vi "Periodic Tasks.vi"(8 "error in":errorcluster) -> ()   [LabVIEW 2018]
doc: "This VI runs in parallel to other robot code. It can contain as many user-defined periodic loops as you need. These can carry out PID or other sorts of timed response."
panel:
  in  "Seconds from neutral to full (0)":sgl=0.08
  out "Transmit FIFO Full Count":u32
  out "Bus Off Count":u32
  out "Percent Bus Utilization":sgl
  out "Receive Error Count":u32
  out "Transmit Error Count":u32
  out "error out":errorcluster
  in  "error in (no error)":errorcluster
  out "Waveform Chart 3":T1(graph)
  out "Waveform Chart 2":T2(graph)
  out "Waveform Chart":dbl(graph)
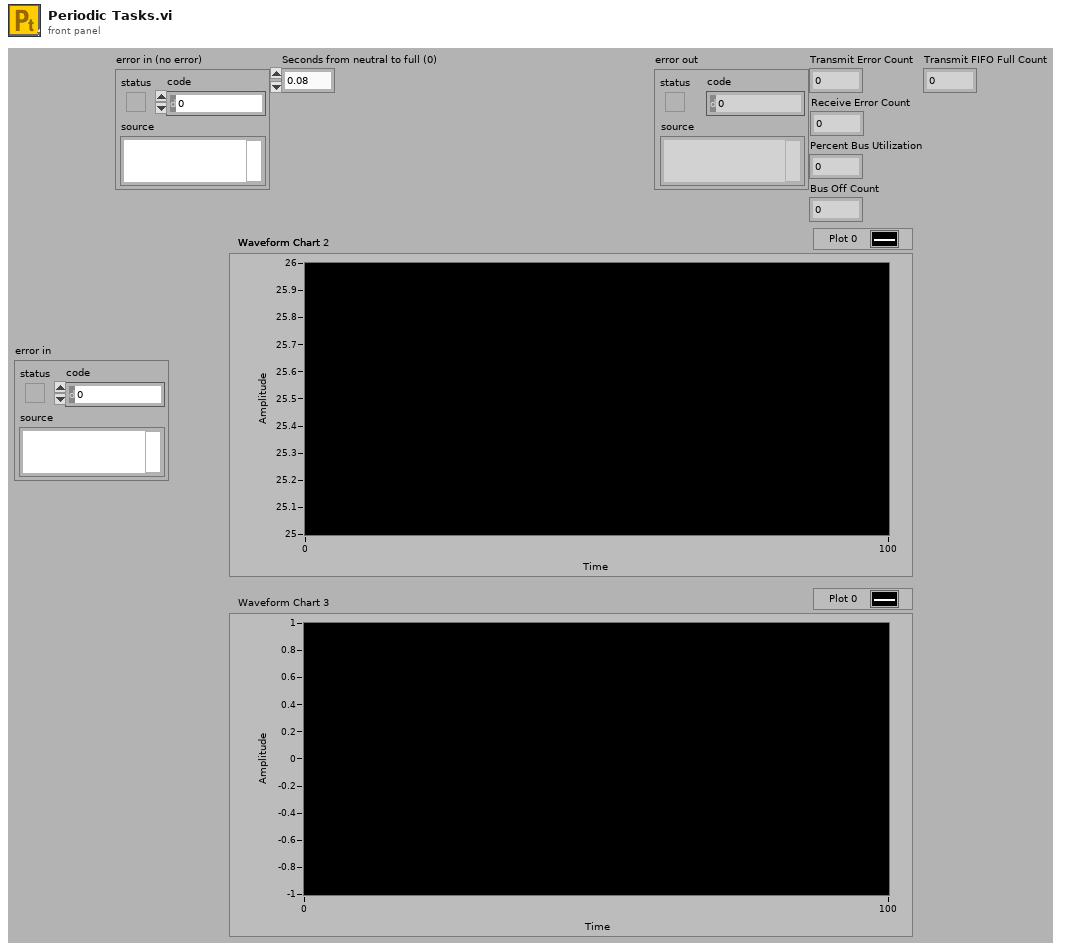
[diagram p1: front panel]
types:
  T1 = cluster{"Sensor Velocity":dbl, "Sensor Velocity":dbl, "Sensor Velocity":dbl}
  T2 = cluster{"Motor Temperature":u8, "Motor Temperature":u8, "Motor Temperature":u8}
  T3 = typedef "SPARKMAX6Motor.ctl" = cluster{"FrontLeftMaster":T4, "FrontLeftSlave1":T4, "FrontLeftSlave2":T4, "FrontRightMaster":T4, "FrontRightSlave1":T4, "FrontRightSlave2":T4}
  T4 = typedef "WPI_MotorControlDeviceRef.ctl" = cluster{"DeviceStatus":errorcluster, "Type":T5, "PWM":cluster{"PWM Channel":T6, "DeadBand":T7}, "CAN":cluster{"Device Number":u8, "SetOutput VI Ref":variant, "GetOutput VI Ref":variant, "Enable VI Ref":variant, "Disable VI Ref":variant, "Data":variant}, "Invert":bool, "DIO PWM":cluster{"PWM \"Enable\" Channel":T6, "DIOChannel":T8, "PWM Rate":dbl}}
  T5 = typedef "WPI_MotorControlType.ctl" = enum16{"PWM", "CAN", "DIO PWM"}
  T6 = typedef "FPGA_DIOPWMChannel.ctl" = enum8{"PWM 0", "PWM 1", "PWM 2", "PWM 3", "PWM 4", "PWM 5", "PWM 6", "PWM 7", "PWM 8", "PWM 9", "PWM MXP 0", "PWM MXP 1", "PWM MXP 2", "PWM MXP 3", "PWM MXP 4", "PWM MXP 5", "PWM MXP 6", "PWM MXP 7", "PWM MXP 8", "PWM MXP 9", "Invalid"}
  T7 = typedef "WPI_PWMDeadband.ctl" = cluster{"Name":string, "maxPositivePwm":i32, "minPositivePwm":i32, "centerPwm":i32, "maxNegativePwm":i32, "minNegativePwm":i32, "angularRange":u16}
  T8 = typedef "FPGA_DIOChannel.ctl" = enum8{"DIO 0", "DIO 1", "DIO 2", "DIO 3", "DIO 4", "DIO 5", "DIO 6", "DIO 7", "DIO 8", "DIO 9", "DIO MXP 0", "DIO MXP 1", "DIO MXP 2", "DIO MXP 3", "DIO MXP 4", "DIO MXP 5", "DIO MXP 6", "DIO MXP 7", "DIO MXP 8", "DIO MXP 9", "DIO MXP 10", "DIO MXP 11", "DIO MXP 12", "DIO MXP 13", "DIO MXP 14", "DIO MXP 15", "SPI Port CS1", "SPI Port CS2", "SPI Port CS3", "SPI Port MISO", "SPI Port MOSI", "Invalid"}
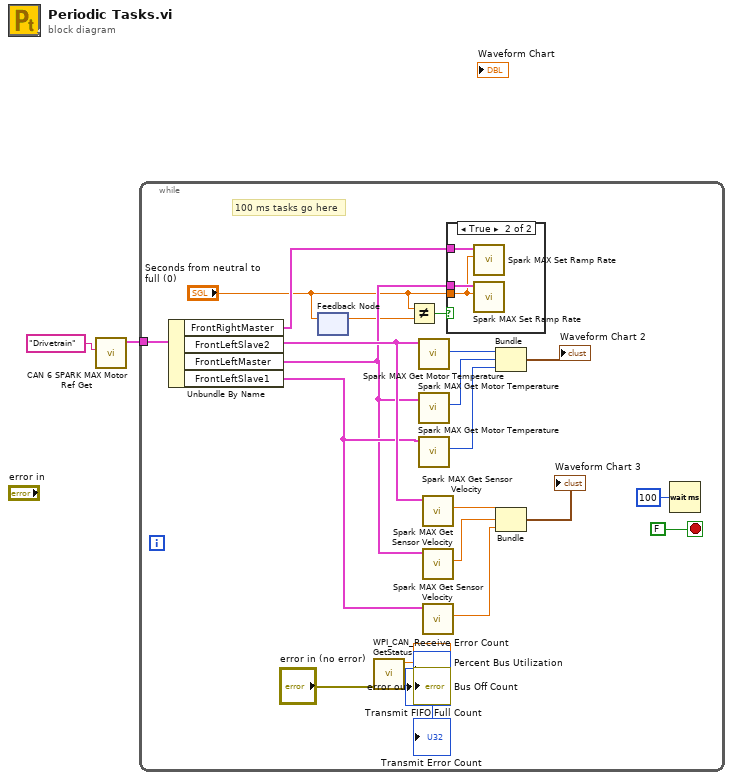
[diagram p0: block diagram]
diagram:
  n1 = call "CAN 6 SPARK MAX Motor Ref Get.vi"("refnum name"="Drivetrain") -> ("TalonSRX6MotorRef out"=w1:T3)  [unwired: 9 in, 1 out]
  n2 = while {
    tunnel: w1 -> [w25]
    stop <- FALSE stop-if-true
    # "100 ms tasks go here"
    n3 = Unbundle By Name(w25) -> ("FrontRightMaster"=w7:T4, "FrontLeftSlave2"=w16:T4, "FrontLeftMaster"=w6:T4, "FrontLeftSlave1"=w15:T4)
    n4 = feedback-in #1("Seconds from neutral to full (0)") -> ()
    n5 = feedback #1() -> (w4:sgl)  [unwired: 1 in]
    n6 = call <vilib>:"WPI_CAN_GetStatus.vi"("error in (no error)"="error in (no error)") -> ("error out"=→"error out":errorcluster, "Transmit Error Count"=→"Transmit Error Count":u32, "Receive Error Count"=→"Receive Error Count":u32, "Percent Bus Utilization"=→"Percent Bus Utilization":sgl, "Bus Off Count"=→"Bus Off Count":u32, "Transmit FIFO Full Count"=→"Transmit FIFO Full Count":u32)  [unwired: 5 in]
    n7 = Not Equal?(x="Seconds from neutral to full (0)", y=w4) -> (x != y?=w5:bool)
    n8 = call <vilib>:"Spark MAX Get Motor Temperature.vi"("MotorControlDevRef in"=w16) -> ("Motor Temperature"=w24:u8)  [unwired: 7 in, 3 out]
    n9 = call <vilib>:"Spark MAX Get Motor Temperature.vi"("MotorControlDevRef in"=w6) -> ("Motor Temperature"=w23:u8)  [unwired: 7 in, 3 out]
    n10 = call <vilib>:"Spark MAX Get Motor Temperature.vi"("MotorControlDevRef in"=w15) -> ("Motor Temperature"=w22:u8)  [unwired: 7 in, 3 out]
    n11 = call <vilib>:"Spark MAX Get Sensor Velocity.vi"("MotorControlDevRef in"=w16) -> ("Sensor Velocity"=w20:dbl)  [unwired: 7 in, 3 out]
    n12 = call <vilib>:"Spark MAX Get Sensor Velocity.vi"("MotorControlDevRef in"=w6) -> ("Sensor Velocity"=w19:dbl)  [unwired: 7 in, 3 out]
    n13 = call <vilib>:"Spark MAX Get Sensor Velocity.vi"("MotorControlDevRef in"=w15) -> ("Sensor Velocity"=w18:dbl)  [unwired: 7 in, 3 out]
    n14 = case shown="True" w5 {
      tunnel: w7 -> [_ w30]
      tunnel: w6 -> [_ w29]
      tunnel: "Seconds from neutral to full (0)" -> [_ w28]
      frame False {
      }
      frame True {
        n15 = call <vilib>:"Spark MAX Set Ramp Rate.vi"("Seconds from neutral to full (0)"=w28, "MotorControlDeviceRef in"=w30) -> ()  [unwired: 8 in, 2 out]
        n16 = call <vilib>:"Spark MAX Set Ramp Rate.vi"("Seconds from neutral to full (0)"=w28, "MotorControlDeviceRef in"=w29) -> ()  [unwired: 8 in, 2 out]
      }
    }
    n17 = Bundle("Motor Temperature"=w24, "Motor Temperature"=w23, "Motor Temperature"=w22) -> (→"Waveform Chart 2":T2)  [unwired: 1 in]
    n18 = Bundle("Sensor Velocity"=w20, "Sensor Velocity"=w19, "Sensor Velocity"=w18) -> (→"Waveform Chart 3":T1)  [unwired: 1 in]
    n19 = Wait (ms)(milliseconds to wait=u32 100) -> ()  [unwired: 1 out]
  }
